vi "Add content to Engine library.vi"(6 "Project Name":string, 8 "error in (no error)":errorcluster, 9 "Project Root":path, 10 "CD Wizard - Internal Data":T1, 11 "CD Template":refnum<class "NIVS_CD Template.lvclass">) -> (0 "error out":errorcluster)   [LabVIEW 2015, in "NIVS_CD Template.lvclass"]
doc: "Add all virtual folders and VIs to the Engine library."
uses:
  NIVS_CD Template.lvclass
  NIVS_Consolidated_CDW_MetaDataObj/Internal data.ctl
  NIVS_Consolidated_CDW_MetaDataObj/CD Engine lvlib.ctl
  NIVS_Consolidated_CDW_MetaDataObj/Add Item - Type.ctl
  NIVS_Consolidated_CDW_MetaDataObj/NIVS_Consolidated_CDW_MetaDataObj.lvclass
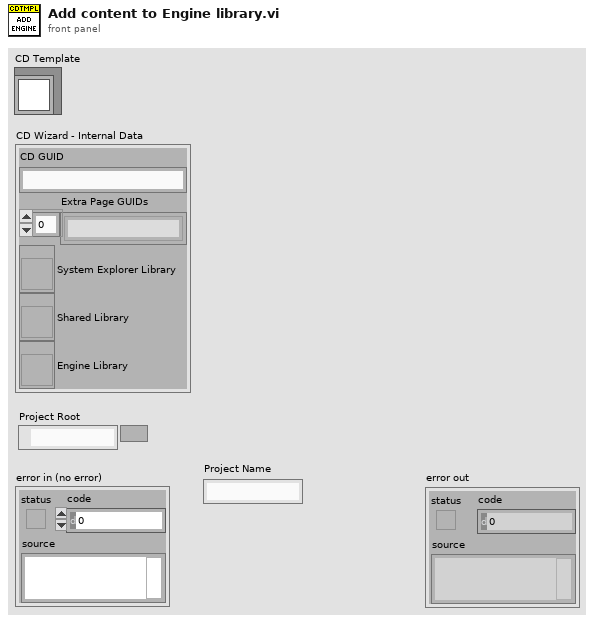
[diagram p1: front panel]
types:
  T1 = typedef "NIVS_Consolidated_CDW_MetaDataObj.lvclass/Internal data.ctl" = cluster{"CD GUID":string, "Extra Page GUIDs":string[], "System Explorer Library":refnum<vi>, "Shared Library":refnum<vi>, "Engine Library":refnum<vi>}
  T2 = typedef "NIVS_Consolidated_CDW_MetaDataObj.lvclass/CD Engine lvlib.ctl" = enum16{"LibraryFileName", "LibraryFolderName", "Engine.FolderName", "Engine.Init.FolderName", "Engine.Run.FolderName", "Engine.Shutdown.FolderName", "Types.FolderName", "Engine.RT Driver VI.TemplatePath", "Engine.RT Driver VI.FileName", "Engine.RTStateVariables.Name", "Engine.RTStateVariables.Name.NoExtension", "Engine.Async.NameExtension", "Engine.Async.TemplateName"}
  T3 = typedef "NIVS_Consolidated_CDW_MetaDataObj.lvclass/Add Item - Type.ctl" = string
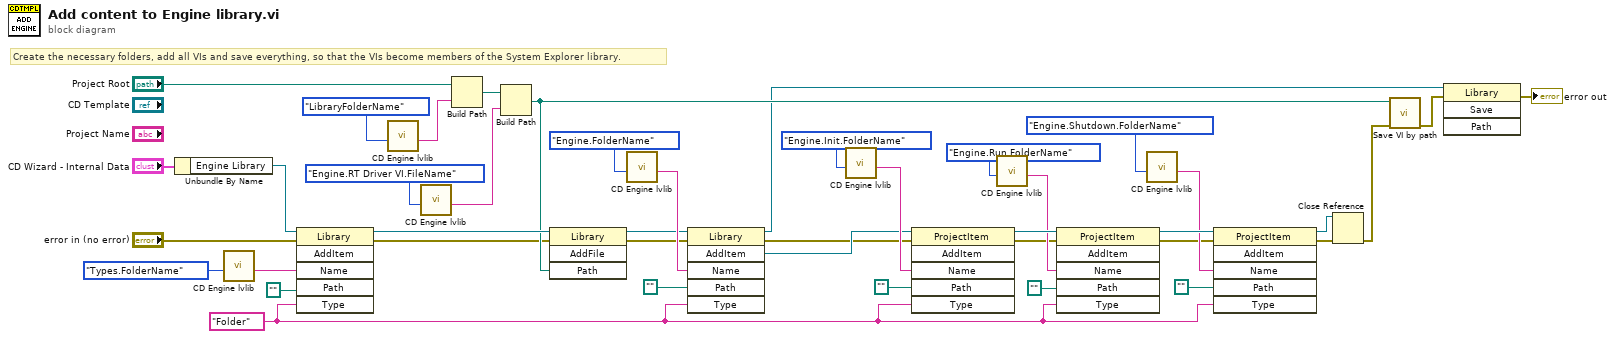
[diagram p0: block diagram]
diagram:
  w13 = T3 "Folder" ("Add Item - Type")
  # "Create the necessary folders, add all VIs and save everything, so that the VIs become members of the System Explorer library."
  n1 = Unbundle By Name("CD Wizard - Internal Data") -> ("Engine Library"=w30:refnum<vi>)
  n2 = call "CD Engine lvlib.vi"("Action"=CD_Engine_lvlib."Types.FolderName") -> ("Output"=w38:string)  [unwired: 10 in]
  n3 = invoke class="Library" method="AddItem"(reference=w30, error in="error in (no error)", "Name"=w38, "Path"=path "", "Type"=w13) -> (reference out=w34:refnum<vi>, error out=w6:errorcluster)  [unwired: 1 in, 4 out]
  n4 = call "CD Engine lvlib.vi"("Action"=CD_Engine_lvlib."LibraryFolderName") -> ("Output"=w32:string)  [unwired: 10 in]
  n5 = call "CD Engine lvlib.vi"("Action"=CD_Engine_lvlib."Engine.RT Driver VI.FileName") -> ("Output"=w33:string)  [unwired: 10 in]
  n6 = Build Path(base path="Project Root", name or relative path=w32) -> (appended path=w31:path)
  n7 = Build Path(base path=w31, name or relative path=w33) -> (appended path=w20:path)
  n8 = invoke class="Library" method="AddFile"(reference=w34, error in=w6, "Path"=w20) -> (reference out=w27:refnum<vi>, error out=w5:errorcluster)  [unwired: 1 in, 2 out]
  n9 = call "CD Engine lvlib.vi"("Action"=CD_Engine_lvlib."Engine.FolderName") -> ("Output"=w28:string)  [unwired: 10 in]
  n10 = invoke class="Library" method="AddItem"(reference=w27, error in=w5, "Name"=w28, "Path"=path "", "Type"=w13) -> (reference out=w19:refnum<vi>, error out=w4:errorcluster, "AddItem"=w26:refnum<vi>)  [unwired: 1 in, 3 out]
  n11 = call "CD Engine lvlib.vi"("Action"=CD_Engine_lvlib."Engine.Init.FolderName") -> ("Output"=w35:string)  [unwired: 10 in]
  n12 = invoke class="ProjectItem" method="AddItem"(reference=w26, error in=w4, "Name"=w35, "Path"=path "", "Type"=w13) -> (reference out=w25:refnum<vi>, error out=w3:errorcluster)  [unwired: 1 in, 4 out]
  n13 = call "CD Engine lvlib.vi"("Action"=CD_Engine_lvlib."Engine.Run.FolderName") -> ("Output"=w24:string)  [unwired: 10 in]
  n14 = invoke class="ProjectItem" method="AddItem"(reference=w25, error in=w3, "Name"=w24, "Path"=path "", "Type"=w13) -> (reference out=w21:refnum<vi>, error out=w2:errorcluster)  [unwired: 1 in, 4 out]
  n15 = call "CD Engine lvlib.vi"("Action"=CD_Engine_lvlib."Engine.Shutdown.FolderName") -> ("Output"=w18:string)  [unwired: 10 in]
  n16 = invoke class="ProjectItem" method="AddItem"(reference=w21, error in=w2, "Name"=w18, "Path"=path "", "Type"=w13) -> (reference out=w15:refnum<vi>, error out=w17:errorcluster)  [unwired: 1 in, 4 out]
  n17 = Close Reference(reference=w15, error in (no error)=w17) -> (error out=w16:errorcluster)
  n18 = call "Save VI by path.vi"("error in (no error)"=w16, "VI path"=w20) -> ("error out"=w39:errorcluster)  [unwired: 9 in]
  n19 = invoke class="Library" method="Save"(reference=w19, error in=w39) -> (error out=→"error out":errorcluster)  [unwired: 2 in, 3 out]
